vi "Hysteresis.vi"(8 "error in":errorcluster, 11 "Book number":i32=375) -> (0 "error out":errorcluster)   [LabVIEW 2021]
uses:
  global.vi
  <vilib>/Utility/file.llb/Write Delimited Spreadsheet (DBL).vi
panel:
  in  "Tab Control":enum32{"Set DAQ", "Source Choice", "Scan"}(tab)=enum."Scan"
  in  "Tab Control 3":enum32{"Fast IV", "Distribution"}(tab)=enum."Distribution"
  in  "Voltage Read":tag="Dev1/ai1"
  in  "samples per channel":i32=2000
  in  "IV Trigger source":tag="/Dev1/PFI12"
  in  "rate":dbl=100000.0 format="%#_13g"
  in  "maximum value":dbl=5.0 format="%#_13g"
  in  "minimum value":dbl format="%#_13g"
  in  "Points per loop":i32=1000
  in  "Box Trigger source":tag="/Dev1/PFI0"
  in  "device in":tag="Dev1"
  in  "Sample Rate":dbl=50.0 format="%.3p"
  in  "Current Read":tag="Dev1/ai2"
  in  "Points Number":i32=10000
  in  "Agi T or SRS F":bool=TRUE
  in  "Field uses Kei  T or DAQ F":bool=TRUE
  in  "Tab Control 2":enum32{"DAQ Field", "Kei Field"}(tab)=enum."Kei Field"
  in  "DAQ Ramp Rate V per s":dbl=0.04
  in  "DAQ Field Out Channel":i32=1
  in  "NI-DAQ Device Number":i32=1
  in  "DAQ Field Read":tag="Dev1/ai3"
  in  "Field Voltage Factor":dbl=2.0 format="%#_13g"
  in  "Init Ramp Time s":dbl=10.0
  in  "Step Ramp Time s":dbl=1.0
  in  "KEITHLEY 2400 GPIB Address":string="13"
  in  "SRS resource name":string="GPIB0::19::INSTR"
  in  "Agi Address":string="GPIB0::10::INSTR"
  in  "Vmax":dbl=6.0
  in  "Frequency Hz":dbl=50.0
  in  "IV or Distribution":bool=TRUE
  in  "Begin field Radius V":dbl=0.5 format="%#_13g"
  in  "Field step V":dbl=0.01 format="%#_13g"
  in  "End field Radius V":dbl=0.5 format="%#_13g"
  out "Current Field mT":dbl=-0.10000000000000009
  out "Current Field V":dbl=-0.010000000000000009
  in  "Field Scale factor":dbl=10.0
  in  "Field Origin V":dbl format="%#_13g"
  in  "Field Radius Step V":dbl=0.008 format="%#_13g"
  in  "Ramp up first T":bool=TRUE
  in  "stop":bool
  in  "Repeat":i32=1
  in  "Ramp type":string(combo)="Around origin"
  in  "Tab Control 4":enum32{"Fast IV", "Distribution"}(tab)=enum."Distribution"
  in  "Current offset uA":dbl=-5.0 format="%#_13g"
  in  "Voltage Amp Scale factor":dbl=0.0005
  in  "Average times":i32=20
  in  "Current step uA":dbl=0.005 format="%#_13g"
  in  "Ic scale factor":dbl=1.0
  in  "Contour plot folder":path=path "C:/Users/gyue/Box Sync/Guang Yue/data/Contour plot"
  # "Field Vread x factor= Field Vapplied"
  # "V_Field*Scale=mT"
  # "Scale * Vread=Vdevice"
  # "Voltage read by DAQ times Scale factor= Ic in uA"
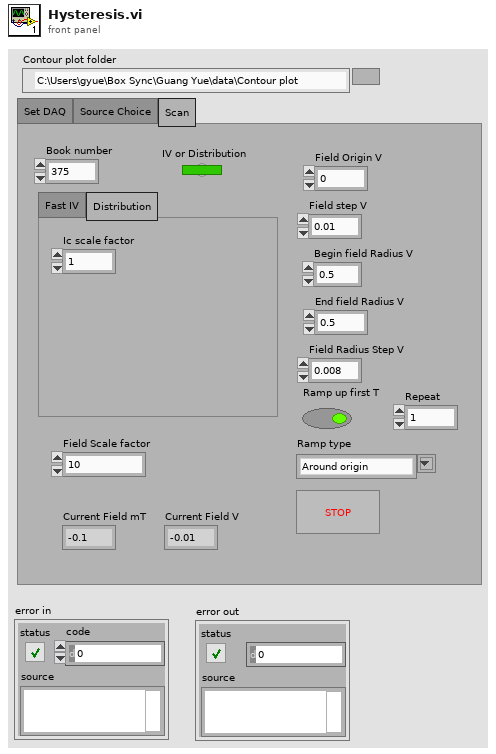
[diagram p1: front panel]
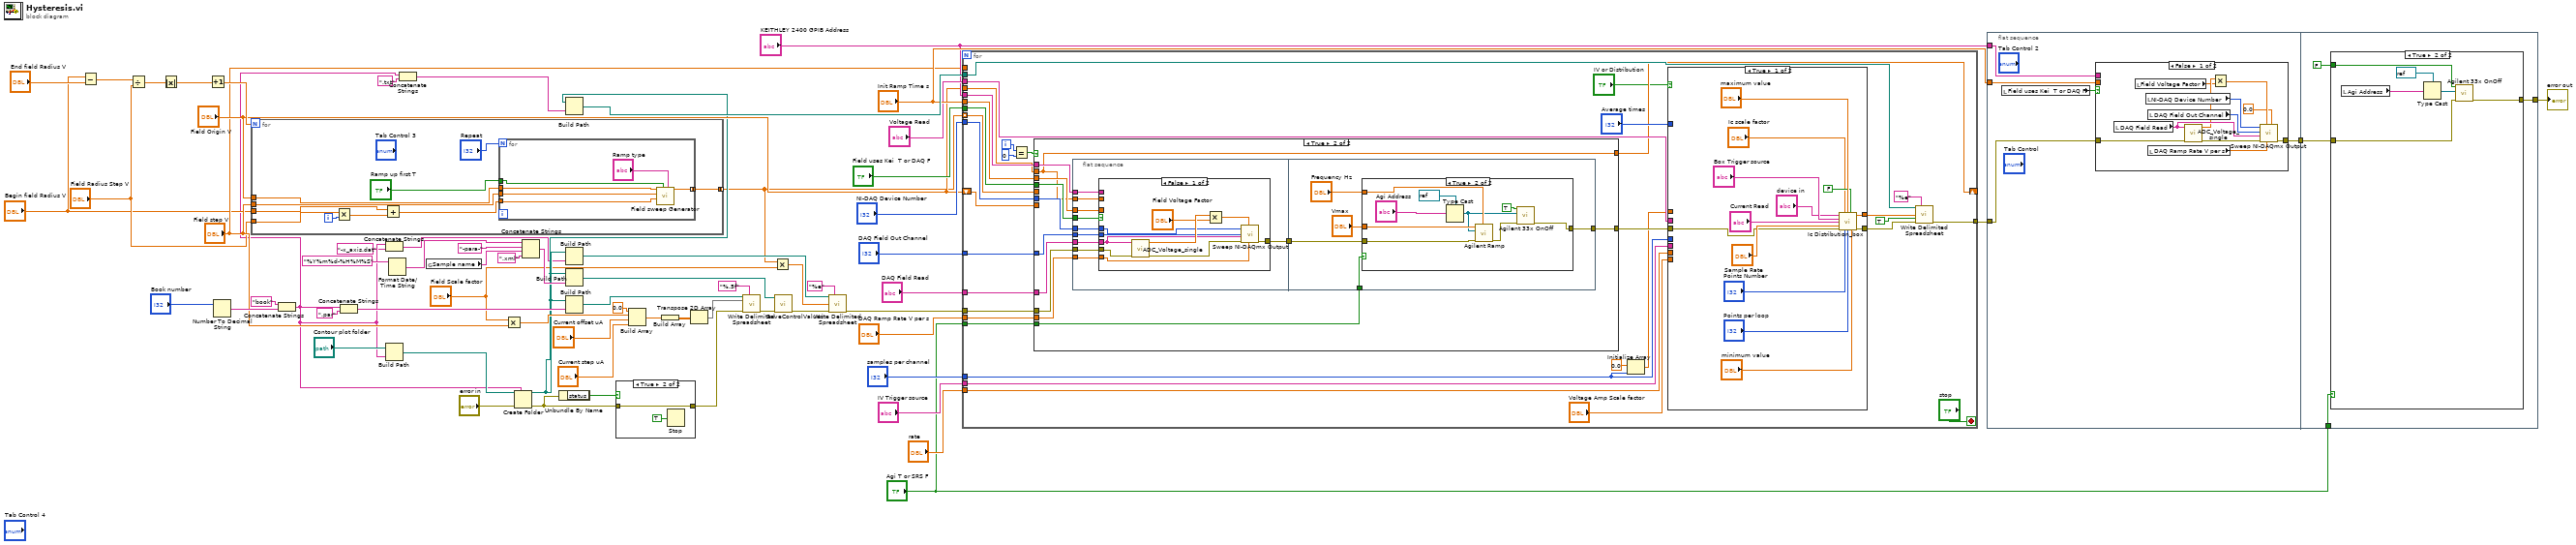
[diagram p0: block diagram]
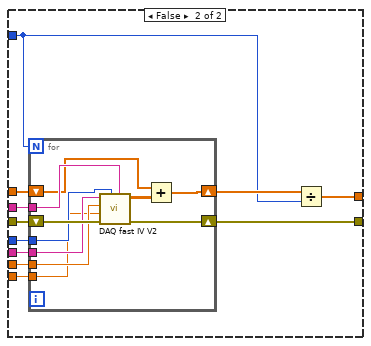
[diagram p2: hidden frame]
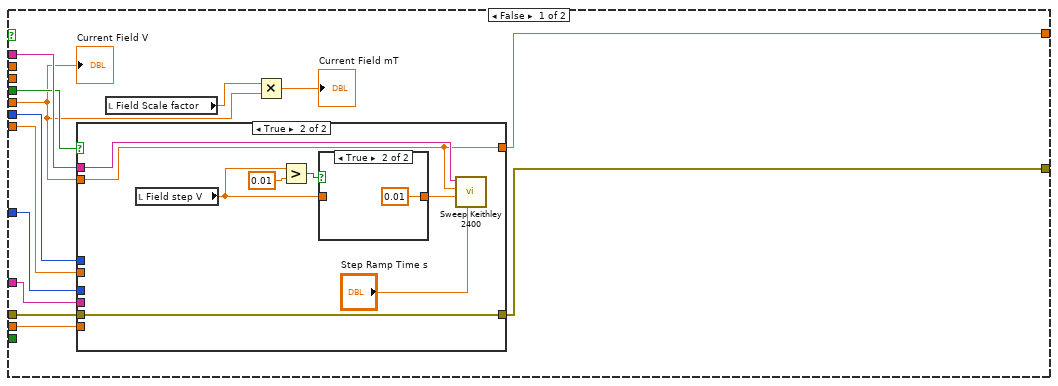
[diagram p3: hidden frame]
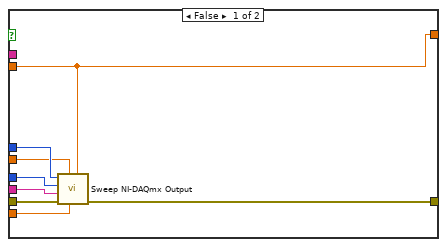
[diagram p4: hidden frame]
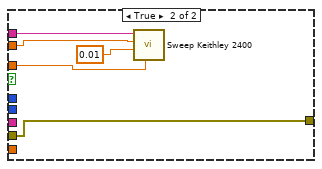
[diagram p6: hidden frame]
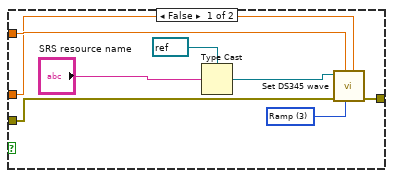
[diagram p7: hidden frame]
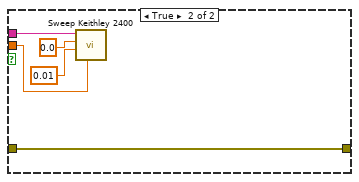
[diagram p8: hidden frame]
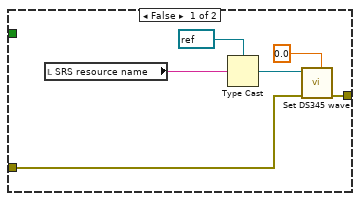
[diagram p9: hidden frame]
diagram:
  n1 = Subtract(x="Begin field Radius V", y="End field Radius V") -> (x-y=w20:dbl)
  n2 = Divide(x=w20, y="Field Radius Step V") -> (x/y=w19:dbl)
  n3 = Absolute Value(x=w19) -> (abs(x)=w18:dbl)
  n4 = Increment(x=w18) -> (x+1=w17:dbl)
  n5 = Number To Decimal String(number="Book number") -> (decimal integer string=w32:string)  [unwired: 1 in]
  n6 = for {
    N: w17 -> [_]
    tunnel: "Field Origin V" -> [w76]
    tunnel: "Field step V" -> [w75]
    tunnel: "Field Radius Step V" -> [w73]
    tunnel: "Begin field Radius V" -> [w71]
    tunnel: [w68] -> w3 mode=concatenating
    i -> [w74]
    n7 = Multiply(x=w73, y=w74) -> (x*y=w72:dbl)
    n8 = Add(x=w71, y=w72) -> (x+y=w70:dbl)
    n9 = for {
      N: "Repeat" -> [_]
      tunnel: w76 -> [w82]
      tunnel: w75 -> [w81]
      tunnel: w70 -> [w80]
      tunnel: "Ramp up first T" -> [w79]
      tunnel: [w78] -> w68 mode=concatenating
      n10 = call "Field sweep Generator.vi"("Ramp type"="Ramp type", "Ramp up first T"=w79, "Field Radius"=w80, "Field step"=w81, "Field Origin"=w82) -> ("output array"=w78:dbl[])  [unwired: 6 in]
    }
  }
  n11 = Concatenate Strings("book" ("string"), w32) -> (w11:string)
  n12 = Concatenate Strings(w11, ".par" ("string")) -> (w60:string)
  n13 = Concatenate Strings(w11, "-x_axis.dat" ("string")) -> (w7:string)
  n14 = Build Path(base path="Contour plot folder", name or relative path=w11) -> (appended path=w50:path)
  n15 = Format Date/Time String(time format string (%c)="%Y%m%d-%H%M%S") -> (date/time string=w12:string)  [unwired: 2 in]
  n16 = Concatenate Strings(w11, ".txt" ("string")) -> (w53:string)
  n17 = global read "global.vi" "Sample name"() -> (w45:string)
  n18 = Multiply(x="Field Scale factor", y="Field step V") -> (x*y=w36:dbl)
  n19 = Create Folder(prompt (Create Folder)=w11, path (use dialog)=w50, error in="error in") -> (created path=w8:path, error out=w47:errorcluster)  [unwired: 1 out]
  n20 = Concatenate Strings(w12, "-para-" ("string"), w45, ".xml" ("string")) -> (w64:string)
  n21 = Unbundle By Name(w47) -> ("status"=w48:bool)
  n22 = Build Path(base path=w8, name or relative path=w53) -> (appended path=w52:path)
  n23 = Build Path(base path=w8, name or relative path=w7) -> (appended path=w6:path)
  n24 = Build Path(base path=w8, name or relative path=w64) -> (appended path=w62:path)
  n25 = Build Path(base path=w8, name or relative path=w60) -> (appended path=w59:path)
  n26 = case shown="True" w48 {
    tunnel: [w83 w85] -> w46
    tunnel: w47 -> [w83 w85]
    frame False {
    }
    frame True {
      n27 = Stop(stop? (T)=TRUE) -> ()
    }
  }
  n28 = Build Array(0.0 ("element"), w36, "Current offset uA", "Current step uA") -> (w57:dbl[])
  n29 = Build Array(w57) -> (w56:dbl[][])
  n30 = Transpose 2D Array(2D array=w56) -> (transposed array=w55:dbl[][])
  n31 = call-poly <vilib>:"Write Delimited Spreadsheet.vi"("file path (dialog if empty)"=w59, "format (%.3f)"="%.5f", "2D data"=w55, "error in (no error)"=w46) -> ("error out"=w49:errorcluster)  [unwired: 10 in, 1 out]
  n32 = Multiply(x=w3, y="Field Scale factor") -> (x*y=w1:dbl[])
  n33 = call "SaveControlValues.vi"("XML File Path"=w62, "error in (no error)"=w49) -> ("error out"=w5:errorcluster)  [unwired: 8 in]
  n34 = call-poly <vilib>:"Write Delimited Spreadsheet.vi"("file path (dialog if empty)"=w6, "format (%.3f)"="%e", "1D data"=w1, "error in (no error)"=w5) -> ("error out"=w4:errorcluster)  [unwired: 10 in, 1 out]
  n35 = for {
    tunnel: "Field step V" -> [_]
    tunnel: w52 -> [w115]
    tunnel: w4 -> [w113]
    tunnel: [w110] -> w44
    tunnel: "Init Ramp Time s" -> [w109]
    tunnel: "Voltage Read" -> [w108]
    tunnel: "samples per channel" -> [w102]
    tunnel: "IV Trigger source" -> [w107]
    tunnel: "rate" -> [w106]
    tunnel: "Agi T or SRS F" -> [w100]
    tunnel: "Field uses Kei  T or DAQ F" -> [w99]
    tunnel: "DAQ Ramp Rate V per s" -> [w98]
    shift-right: [w89] -> _
    shift-left: "Field Origin V" -> [w97]
    tunnel: "NI-DAQ Device Number" -> [w94]
    tunnel: "DAQ Field Out Channel" -> [w93]
    tunnel: "KEITHLEY 2400 GPIB Address" -> [w92]
    tunnel: "DAQ Field Read" -> [w91]
    tunnel: "Field Origin V" -> [w90]
    tunnel: w3 -> [w88] mode=indexing
    i -> [w96]
    stop <- "stop" stop-if-true
    n36 = Equal?(x=w96, y=0) -> (x = y?=w114:bool)
    n37 = case shown="True" w114 {
      tunnel: w113 -> [w163 w193]
      tunnel: [w162 w192] -> w112
      tunnel: w92 -> [w165 w195]
      tunnel: w109 -> [_ w191]
      tunnel: w100 -> [_ w190]
      tunnel: w99 -> [w164 w189]
      tunnel: w98 -> [w161 w188]
      tunnel: w93 -> [w159 w187]
      tunnel: w94 -> [w160 w186]
      tunnel: w91 -> [w158 w185]
      tunnel: w97 -> [w157 _]
      tunnel: w90 -> [_ w184]
      tunnel: [w156 w184] -> w89
      tunnel: w88 -> [w154 _]
      frame False {
        n38 = case shown="True" w164 {
          tunnel: w165 -> [_ w176]
          tunnel: w163 -> [w173 w175]
          tunnel: [w172 w175] -> w162
          tunnel: w161 -> [w171 _]
          tunnel: w160 -> [w170 _]
          tunnel: w159 -> [w169 _]
          tunnel: w158 -> [w168 _]
          tunnel: w157 -> [w167 _]
          tunnel: w154 -> [w166 w174]
          tunnel: [w166 w174] -> w156
          frame False {
            n39 = call "Sweep NI-DAQmx Output.vi"("Final Output Value"=w166, "Ramp Rate V/s"=w171, "Init Input Voltage"=w167, "error in"=w173, "Field Read Voltage"=w168, "Output Channel"=w169, "NI-DAQ Device Number"=w170) -> ("error out"=w172:errorcluster)  [unwired: 4 in]
          }
          frame True {
            n40 = local read "Field step V"() -> (w177:dbl)
            n41 = Greater?(x=w177, y=0.01) -> (0:w179:bool)
            n42 = case shown="True" w179 {
              tunnel: [w182 0.01 ("Gate Step [V]")] -> w178
              tunnel: w177 -> [w182 _]
              frame False {
              }
              frame True {
              }
            }
            n43 = call "Sweep Keithley 2400.vi"("Ramp Time (s)"="Step Ramp Time s", "Gate Step [V]"=w178, "final gate voltage (V)"=w174, "KEITHLEY 2400 GPIB Address"=w176) -> ()  [unwired: 6 in, 2 out]
          }
        }
        n44 = local read "Field Scale factor"() -> (w155:dbl)
        n45 = Multiply(x=w155, y=w154) -> (x*y=→"Current Field mT":dbl)
        "Current Field V" <- w154
      }
      frame True {
        n46 = flat-sequence {
          tunnel: w195 -> [w205]
          tunnel: [w201] -> w194
          tunnel: w193 -> [w202]
          tunnel: w191 -> [w204]
          tunnel: w189 -> [w203]
          tunnel: w188 -> [w200]
          tunnel: w187 -> [w199]
          tunnel: w186 -> [w198]
          tunnel: w185 -> [w197]
          tunnel: w184 -> [w196]
          tunnel: w194 -> [w225]
          tunnel: [w224] -> w192
          tunnel: w190 -> [w221]
          frame #0 {
            n47 = case shown="False" w203 {
              tunnel: w205 -> [_ w220]
              tunnel: w204 -> [_ w219]
              tunnel: w202 -> [w211 w217]
              tunnel: [w210 w217] -> w201
              tunnel: w200 -> [w209 _]
              tunnel: w199 -> [w208 _]
              tunnel: w198 -> [w207 _]
              tunnel: w197 -> [w206 _]
              tunnel: w196 -> [_ w216]
              frame False {
                n48 = call "ADC_Voltage_single.vi"("error in"=w211, "physical channels"=w206) -> ("error out"=w215:errorcluster, "data"=w214:dbl)  [unwired: 8 in]
                n49 = Multiply(x=w214, y="Field Voltage Factor") -> (x*y=w212:dbl)
                n50 = call "Sweep NI-DAQmx Output.vi"("Ramp Rate V/s"=w209, "Init Input Voltage"=w212, "error in"=w215, "Field Read Voltage"=w206, "Output Channel"=w208, "NI-DAQ Device Number"=w207) -> ("error out"=w210:errorcluster)  [unwired: 5 in]
              }
              frame True {
                n51 = call "Sweep Keithley 2400.vi"("Ramp Time (s)"=w219, "Gate Step [V]"=0.01, "final gate voltage (V)"=w216, "KEITHLEY 2400 GPIB Address"=w220) -> ()  [unwired: 6 in, 2 out]
              }
            }
          }
          frame #1 {
            n52 = case shown="True" w221 {
              tunnel: w225 -> [w233 w242]
              tunnel: [w232 w240] -> w224
              tunnel: "Vmax" -> [w229 w238]
              tunnel: "Frequency Hz" -> [w230 w237]
              frame False {
                w231 = u16 3 items=["Sine", "Square", "Triangle", "Ramp", "Noise"] ("Waveform Function (0: Sine)")
                n53 = Type Cast(type=refnum<visa-resource-name> refnum ("SRS resource name 2"), x="SRS resource name") -> (*(type *) &x=w226:refnum<visa-resource-name>)
                n54 = call "Set DS345 wave.vi"("Amplitude (0.01 Vpp)"=w229, "Waveform Function (0: Sine)"=w231, "Frequency (1000 Hz)"=w230, "error in (no error)"=w233, "VISA resource name"=w226) -> ("error out"=w232:errorcluster)  [unwired: 6 in]
              }
              frame True {
                n55 = Type Cast(type=refnum<visa-resource-name> refnum ("SRS resource name 2"), x="Agi Address") -> (*(type *) &x=w234:refnum<visa-resource-name>)
                n56 = call "Agilent Ramp.vi"("Frequency Hz"=w237, "error in (no error)"=w242, "VISA resource name"=w234, "Vmax"=w238) -> ("error out"=w241:errorcluster)  [unwired: 7 in]
                n57 = call "Agilent 33x OnOff.vi"("error in (no error)"=w241, "VISA resource name"=w234, "Enable Output  (T: Enable)"=TRUE) -> ("error out"=w240:errorcluster)  [unwired: 8 in]
              }
            }
          }
        }
      }
    }
    n58 = Initialize Array(0.0 ("element"), w102) -> (w101:dbl[])
    n59 = case shown="True" "IV or Distribution" {
      tunnel: w112 -> [w119 w142]
      tunnel: [w121 w141] -> w111
      tunnel: w108 -> [_ w140]
      tunnel: w107 -> [_ w139]
      tunnel: w106 -> [_ w138]
      tunnel: "Average times" -> [_ w136]
      tunnel: [w122 w135] -> w104
      tunnel: w102 -> [_ w134]
      tunnel: w101 -> [_ w133]
      tunnel: "Voltage Amp Scale factor" -> [_ w132]
      frame True {
        n60 = call "Ic Distribution_box.vi"("device in"="device in", "Scale factor"="Ic scale factor", "maximum value"="maximum value", "Log Data"=FALSE, "Trigger source"="Box Trigger source", "Current Read"="Current Read", "Sample Rate"="Sample Rate", "error in no error"=w119, "Points Number"="Points Number", "Points per loop"="Points per loop", "minimum value"="minimum value") -> ("Ic array"=w122:dbl[], "error out"=w121:errorcluster)  [unwired: 3 in]
      }
      frame False {
        n61 = for {
          N: w136 -> [_]
          tunnel: w140 -> [w150]
          tunnel: w134 -> [w149]
          tunnel: w139 -> [w148]
          tunnel: w138 -> [w147]
          shift-right: [w151] -> w141
          shift-left: w142 -> [w152]
          shift-right: [w145] -> w137
          shift-left: w133 -> [w144]
          tunnel: w132 -> [w143]
          n62 = call "DAQ fast IV V2.vi"("physical channels I and V"=w150, "samples per channel"=w149, "error in"=w152, 9:w143, "rate"=w147, "Trigger source"=w148) -> ("error out"=w151:errorcluster, "Output"=w146:dbl[][])  [unwired: 4 in]
          n63 = Add(x=w144, y=w146) -> (x+y=w145:dbl[])
        }
        n64 = Divide(x=w137, y=w136) -> (x/y=w135:dbl[])
      }
    }
    n65 = call-poly <vilib>:"Write Delimited Spreadsheet.vi"("file path (dialog if empty)"=w115, "format (%.3f)"="%e", "1D data"=w104, "append to file? (new file:F)"=TRUE ("append to file? (F)"), "error in (no error)"=w111) -> ("error out"=w110:errorcluster)  [unwired: 9 in, 1 out]
  }
  n66 = flat-sequence {
    tunnel: w44 -> [w244]
    tunnel: "KEITHLEY 2400 GPIB Address" -> [w247]
    tunnel: [w243] -> w42
    tunnel: "Init Ramp Time s" -> [w246]
    tunnel: [w266] -> w43
    tunnel: w42 -> [w267]
    tunnel: "Agi T or SRS F" -> [w264]
    frame #0 {
      n67 = local read "Field uses Kei  T or DAQ F"() -> (w245:bool)
      n68 = case shown="False" w245 {
        tunnel: w247 -> [_ w262]
        tunnel: w246 -> [_ w261]
        tunnel: w244 -> [w250 w259]
        tunnel: [w249 w259] -> w243
        frame False {
          n69 = local read "DAQ Field Read"() -> (w255:tag)
          n70 = local read "Field Voltage Factor"() -> (w248:dbl)
          n71 = local read "NI-DAQ Device Number"() -> (w256:i32)
          n72 = local read "DAQ Field Out Channel"() -> (w257:i32)
          n73 = local read "DAQ Ramp Rate V per s"() -> (w258:dbl)
          n74 = call "ADC_Voltage_single.vi"("error in"=w250, "physical channels"=w255) -> ("error out"=w252:errorcluster, "data"=w253:dbl)  [unwired: 8 in]
          n75 = Multiply(x=w253, y=w248) -> (x*y=w254:dbl)
          n76 = call "Sweep NI-DAQmx Output.vi"("Final Output Value"=0.0, "Ramp Rate V/s"=w258, "Init Input Voltage"=w254, "error in"=w252, "Field Read Voltage"=w255, "Output Channel"=w257, "NI-DAQ Device Number"=w256) -> ("error out"=w249:errorcluster)  [unwired: 4 in]
        }
        frame True {
          n77 = call "Sweep Keithley 2400.vi"("Ramp Time (s)"=w261, "Gate Step [V]"=0.01, "final gate voltage (V)"=0.0, "KEITHLEY 2400 GPIB Address"=w262) -> ()  [unwired: 6 in, 2 out]
        }
      }
    }
    frame #1 {
      n78 = case shown="True" w264 {
        tunnel: w267 -> [w273 w279]
        tunnel: [w272 w278] -> w266
        tunnel: FALSE ("Enable Output  (T: Enable)") -> [_ w277]
        frame False {
          n79 = local read "SRS resource name"() -> (w268:string)
          n80 = Type Cast(type=refnum<visa-resource-name> refnum ("SRS resource name 2"), x=w268) -> (*(type *) &x=w269:refnum<visa-resource-name>)
          n81 = call "Set DS345 wave.vi"("Amplitude (0.01 Vpp)"=0.0, "error in (no error)"=w273, "VISA resource name"=w269) -> ("error out"=w272:errorcluster)  [unwired: 8 in]
        }
        frame True {
          n82 = local read "Agi Address"() -> (w275:string)
          n83 = Type Cast(type=refnum<visa-resource-name> refnum ("SRS resource name 2"), x=w275) -> (*(type *) &x=w274:refnum<visa-resource-name>)
          n84 = call "Agilent 33x OnOff.vi"("error in (no error)"=w279, "VISA resource name"=w274, "Enable Output  (T: Enable)"=w277) -> ("error out"=w278:errorcluster)  [unwired: 8 in]
        }
      }
    }
  }
  "error out" <- w43
